vi "Toggle Alpha Blending.vi"(11 "Scene in":refnum<class "Scene.lvclass">) -> (3 "Scene out":refnum<class "Scene.lvclass">)   [LabVIEW 2022 SP3, in "Application.lvlib" / "Scene.lvclass"]
uses:
  Scene.lvclass
  Scene.lvclass/Scene.ctl
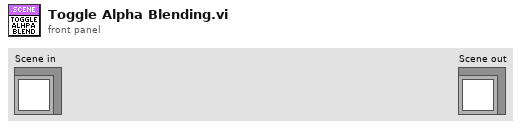
[diagram p1: front panel]
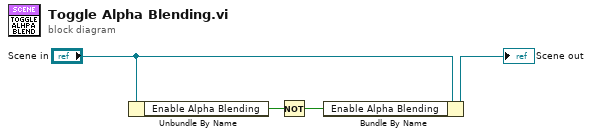
[diagram p0: block diagram]
diagram:
  n1 = Unbundle By Name("Scene in") -> ("Enable Alpha Blending"=w3:bool)
  n2 = Not(x=w3) -> (.not. x?=w4:bool)
  n3 = Bundle By Name(cluster="Scene in", "Enable Alpha Blending"=w4) -> (→"Scene out":refnum<class "Scene.lvclass">)
